vi "Wavelength iHR320.vi"(8 "error in (no error)":errorcluster, 10 "Spectrometer iHR320.lvclass":refnum<class "Spectrometer iHR320.lvclass">, 11 "Wavelength iHR320.lvclass In":refnum<class "Wavelength iHR320.lvclass">) -> (0 "error out":errorcluster, 3 "Wavelength iHR320.lvclass Out":refnum<class "Wavelength iHR320.lvclass">)   [LabVIEW 2009, in "Wavelength iHR320.lvclass"]
uses:
  Wavelength iHR320.lvclass
  Instruments/Spectrometer iHR320/Spectrometer iHR320.lvclass
  Global/GPIB Numbers.vi
  Wavelength iHR320.lvclass/Wavelength iHR320.ctl
  Scanner/Scanner.lvclass
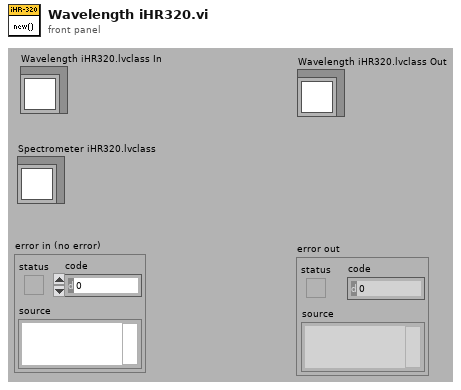
[diagram p1: front panel]
types:
  T1 = typedef "USBMono Type Def.ctl" = cluster{"Name":string, "Unique ID":string, "FW Unique ID":string}
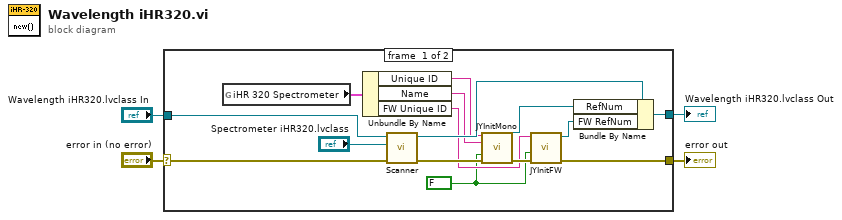
[diagram p0: block diagram]
diagram:
  n1 = case shown="No Error" "error in (no error)" {
    selector: "error in (no error)" -> [w17 w20]
    tunnel: [w8 w20] -> w3
    tunnel: "Wavelength iHR320.lvclass In" -> [w19 w21]
    tunnel: [w14 w21] -> w1
    frame #0 {
      w6 = FALSE ("Force Init")
      n2 = global read "GPIB Numbers.vi" "iHR 320 Spectrometer"() -> (w15:T1)
      n3 = Unbundle By Name(w15) -> ("Unique ID"=w11:string, "Name"=w10:string, "FW Unique ID"=w7:string)
      n4 = call "Scanner.vi"("error in (no error)"=w17, "Scannable"="Spectrometer iHR320.lvclass", "Scanner.lvclass in"=w19) -> ("error out"=w13:errorcluster, "Scanner.lvclass out"=w16:refnum<class "Wavelength iHR320.lvclass">)  [unwired: 7 in]
      n5 = call "JYInitMono.vi"("Unique ID"=w11, "Mono ID"=w10, "Force Init"=w6, "error in (no error)"=w13) -> ("Mono RefNum out"=w12:refnum<k7>, "error out"=w9:errorcluster)  [unwired: 7 in, 3 out]
      n6 = call "JYInitFW.vi"("error in (no error)"=w9, "Force?"=w6, "FW Unique ID"=w7) -> ("error out"=w8:errorcluster, "FW RefNum Out"=w5:refnum<k7>)  [unwired: 5 in, 2 out]
      n7 = Bundle By Name(cluster=w16, "RefNum"=w12, "FW RefNum"=w5) -> (w14:refnum<class "Wavelength iHR320.lvclass">)
    }
    frame #1 {
    }
  }
  "error out" <- w3
  "Wavelength iHR320.lvclass Out" <- w1
